vi "After Launch Init Core.vi"(8 "error in (no error)":errorcluster, 11 "CS++Motor in":refnum<class "CS++Motor.lvclass">) -> (0 "error out":errorcluster, 3 "CS++Motor out":refnum<class "CS++Motor.lvclass">)   [LabVIEW 2016, in "CS++Motor.lvlib" / "CS++Motor.lvclass"]
doc: "Use <b>Pre Launch init.vi</b> method for sanity checks that are supposed to prevent the actor from launching if they fail. Use <B>this</B> method instead to initialize this actor when it has been activated. A corresponding high priority message will become dispatched before the <B>Actor Core.vi</b> is called.\n\n<b>Derived classed should call the parent methode first</b> and their own initialization code after.\n\nRefer also to the ongoing discussion at https://decibel.ni.com/content/message/57394#57394."
uses:
  CS++Motor.lvclass
  C:/Program Files (x86)/National Instruments/LabVIEW 2016/vi.lib/ActorFramework/Actor/Actor.lvclass
  CSPP_Core/Classes/CS++ProcessVariables/ProcessVariable/PV.lvclass
  CS++Motor.lvclass/CS++Motor.ctl
  CSPP_Core/Classes/CS++ProcessVariables/ProcessVariable/PV.lvclass/PV.ctl
  <vilib>/ActorFramework/Actor/Actor.lvclass/Actor.ctl
  <vilib>/ActorFramework/Message Enqueuer/Message Enqueuer.lvclass/Message Enqueuer.ctl
  CSPP_Core/Actors/CS++DeviceActor Messages/Reset Device Msg/Reset Device Msg.lvclass/Reset Device Msg.ctl
  CSPP_Core/Classes/CS++ProcessVariables/ProcessVariable/Write Data.vi
  CSPP_Core/Classes/CS++ProcessVariables/ProcessVariable/Write Error.vi
  CSPP_Core/Classes/CS++ProcessVariables/ProcessVariable/Write Quality.vi
  CSPP_Core/Classes/CS++ProcessVariables/ProcessVariable/Write status.vi
  CSPP_Core/Classes/CS++ProcessVariables/ProcessVariable/Write Timestamp.vi
  <vilib>/ActorFramework/Message Enqueuer/Init from Existing Queue.vi
  <vilib>/ActorFramework/Message Enqueuer/Enqueue.vi
  CSPP_Core/Actors/CS++DeviceActor Messages/Reset Device Msg/Reset Device Msg.lvclass
  C:/Program Files (x86)/National Instruments/LabVIEW 2016/vi.lib/ActorFramework/Message/Message.lvclass
  <vilib>/ActorFramework/Message Priority Queue/Priority Enqueue.vi
  <vilib>/ActorFramework/Message Enqueuer/Message Enqueuer.lvclass
  CSPP_Core/Actors/CS++DeviceActor/CS++DeviceActor.lvclass
  CSPP_Core/Classes/CS++ProcessVariables/PVConnection/PVConnection.lvclass
  <vilib>/ActorFramework/Actor/Actor.lvclass
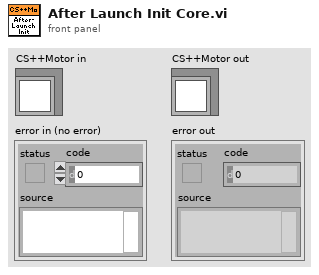
[diagram p1: front panel]
types:
  T1 = cluster{"Read Access":enum8{"Allowed", "Required", "None"}, "Write Access":enum8{"Allowed", "Required", "None"}}
  T2 = cluster{"LogicalName":string, "PhysicalName":string, "unit":string, "Scaling":dbl, "Scaling Offset":dbl, "StartVelocity":dbl, "StopVelocity":dbl, "Acceleration":dbl, "RangeMin":dbl, "RangeMax":dbl, "LogicalPos-Array":cluster{"LogicalPosition":string, "SetPosition":dbl}[]}[]
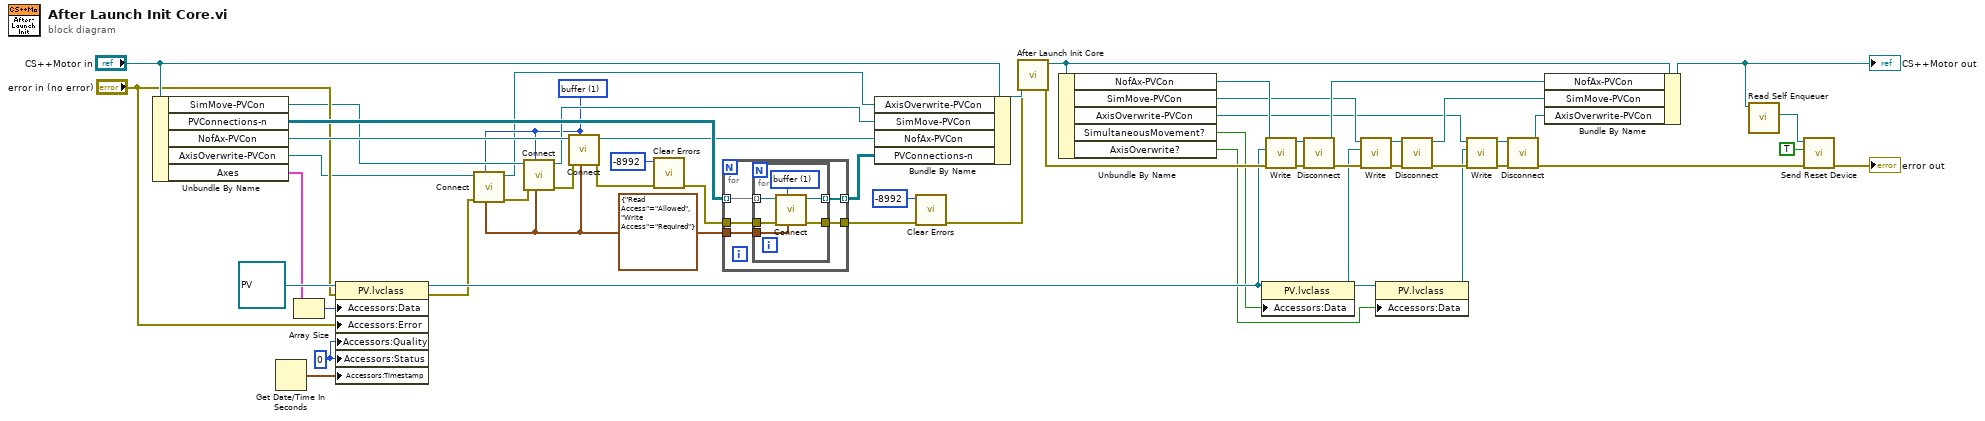
[diagram p0: block diagram]
diagram:
  w9 = u16 1 items=["commit", "buffer"] ("Mode (commit)")
  w8 = T1 {"Read Access"=enum."Allowed", "Write Access"=enum."Required"} ("Access (R/W allowed)")
  w52 = 0 ("Quality")
  n1 = Unbundle By Name("CS++Motor in") -> ("SimMove-PVCon"=w29:refnum<class "PVConnection.lvclass">, "PVConnections-n"=w47:refnum<class "PVConnection.lvclass">[][], "NofAx-PVCon"=w49:refnum<class "PVConnection.lvclass">, "AxisOverwrite-PVCon"=w7:refnum<class "PVConnection.lvclass">, "Axes"=w12:T2)
  n2 = Get Date/Time In Seconds() -> (seconds since 1Jan1904=w53:timestamp)
  n3 = Array Size(array=w12) -> (size(s)=w51:i32)
  n4 = property class="PV.lvclass"(reference=refnum<class "PV.lvclass"> refnum ("CS++ProcessVariables.lvlib:PV.lvclass"), error in="error in (no error)", "Accessors:Data"=w51, "Accessors:Error"="error in (no error)", "Accessors:Quality"=w52, "Accessors:Status"=w52, "Accessors:Timestamp"=w53) -> (reference out=w27:refnum<class "PV.lvclass">, error out=w11:errorcluster)
  n5 = call "Connect.vi"("Access (R/W allowed)"=w8, "Mode (buffer)"=w9, "Error In"=w11, "PVConnection in"=w7) -> ("Error Out"=w10:errorcluster, "PVConnection out"=w6:refnum<class "PVConnection.lvclass">)  [unwired: 6 in]
  n6 = call "Connect.vi"("Access (R/W allowed)"=w8, "Mode (buffer)"=w9, "Error In"=w10, "PVConnection in"=w29) -> ("Error Out"=w30:errorcluster, "PVConnection out"=w28:refnum<class "PVConnection.lvclass">)  [unwired: 6 in]
  n7 = call "Connect.vi"("Access (R/W allowed)"=w8, "Mode (buffer)"=w9, "Error In"=w30, "PVConnection in"=w49) -> ("Error Out"=w40:errorcluster, "PVConnection out"=w43:refnum<class "PVConnection.lvclass">)  [unwired: 6 in]
  n8 = call <vilib>:"Clear Errors.vi"("error in (no error)"=w40, "specific error code to clear (0: all)"=-8992) -> ("error out"=w31:errorcluster)  [unwired: 4 in, 1 out]
  n9 = for {
    tunnel: w8 -> [w58]
    tunnel: w47 -> [w57] mode=indexing
    tunnel: [w56] -> w46 mode=indexing
    tunnel: w31 -> [w54]
    tunnel: [w55] -> w45
    n10 = for {
      tunnel: w57 -> [w64] mode=indexing
      tunnel: [w63] -> w56 mode=indexing
      tunnel: w58 -> [w62]
      tunnel: [w61] -> w55
      tunnel: w54 -> [w59]
      w60 = u16 1 items=["commit", "buffer"] ("Mode (commit)")
      n11 = call "Connect.vi"("Access (R/W allowed)"=w62, "Mode (buffer)"=w60, "Error In"=w59, "PVConnection in"=w64) -> ("Error Out"=w61:errorcluster, "PVConnection out"=w63:refnum<class "PVConnection.lvclass">)  [unwired: 6 in]
    }
  }
  n12 = Bundle By Name(cluster="CS++Motor in", "AxisOverwrite-PVCon"=w6, "SimMove-PVCon"=w28, "NofAx-PVCon"=w43, "PVConnections-n"=w46) -> (w48:refnum<class "CS++Motor.lvclass">)
  n13 = call <vilib>:"Clear Errors.vi"("error in (no error)"=w45, "specific error code to clear (0: all)"=-8992) -> ("error out"=w42:errorcluster)  [unwired: 4 in, 1 out]
  n14 = call-parent "After Launch Init Core.vi"("error in (no error)"=w42, "CS++DeviceActor in"=w48) -> ("error out"=w35:errorcluster, "CS++DeviceActor out"=w39:refnum<class "CS++Motor.lvclass">)  [unwired: 8 in]
  n15 = Unbundle By Name(w39) -> ("NofAx-PVCon"=w37:refnum<class "PVConnection.lvclass">, "SimMove-PVCon"=w25:refnum<class "PVConnection.lvclass">, "AxisOverwrite-PVCon"=w14:refnum<class "PVConnection.lvclass">, "SimultaneousMovement?"=w21:bool, "AxisOverwrite?"=w13:bool)
  n16 = property class="PV.lvclass"(reference=w27, "Accessors:Data"=w21) -> (reference out=w16:refnum<class "PV.lvclass">)  [unwired: 1 in, 1 out]
  n17 = call "Write.vi"("error in (no error)"=w35, "PV"=w27, "PVConnection in"=w37) -> ("error out"=w36:errorcluster, "PVConnection out"=w38:refnum<class "PVConnection.lvclass">)  [unwired: 7 in]
  n18 = call "Disconnect.vi"("error in (no error)"=w36, "PVConnection in"=w38) -> ("error out"=w26:errorcluster, "PVConnection out"=w34:refnum<class "PVConnection.lvclass">)  [unwired: 8 in]
  n19 = call "Write.vi"("error in (no error)"=w26, "PV"=w16, "PVConnection in"=w25) -> ("error out"=w24:errorcluster, "PVConnection out"=w23:refnum<class "PVConnection.lvclass">)  [unwired: 7 in]
  n20 = property class="PV.lvclass"(reference=w16, "Accessors:Data"=w13) -> (reference out=w15:refnum<class "PV.lvclass">)  [unwired: 1 in, 1 out]
  n21 = call "Disconnect.vi"("error in (no error)"=w24, "PVConnection in"=w23) -> ("error out"=w18:errorcluster, "PVConnection out"=w22:refnum<class "PVConnection.lvclass">)  [unwired: 8 in]
  n22 = call "Write.vi"("error in (no error)"=w18, "PV"=w15, "PVConnection in"=w14) -> ("error out"=w19:errorcluster, "PVConnection out"=w20:refnum<class "PVConnection.lvclass">)  [unwired: 7 in]
  n23 = call "Disconnect.vi"("error in (no error)"=w19, "PVConnection in"=w20) -> ("error out"=w2:errorcluster, "PVConnection out"=w17:refnum<class "PVConnection.lvclass">)  [unwired: 8 in]
  n24 = Bundle By Name(cluster=w39, "NofAx-PVCon"=w34, "SimMove-PVCon"=w22, "AxisOverwrite-PVCon"=w17) -> (w3:refnum<class "CS++Motor.lvclass">)
  "CS++Motor out" <- w3
  n25 = call <vilib>:"Read Self Enqueuer.vi"("Actor"=w3) -> ("Self Enqueuer"=w5:refnum<class "Message Enqueuer.lvclass">)  [unwired: 10 in]
  n26 = call "Send Reset Device.vi"("error in (no error)"=w2, "Reset"=TRUE, "Message Enqueuer"=w5) -> ("error out"=→"error out":errorcluster)  [unwired: 7 in, 1 out]
